vi "Terminate.vi"(8 "error in (no error)":errorcluster, 10 "Message in":refnum<class "TerminateMessage.lvclass">, 11 "ImageStack in":refnum<class "Invivo_ImageStack.lvclass">) -> (0 "error out":errorcluster, 3 "ImageStack out":refnum<class "Invivo_ImageStack.lvclass">)   [LabVIEW 2012, in "Invivo_ImageStack.lvclass"]
doc: "This member function is called when the statemachine in the run.vi receives an 'terminate' command. It closes the RabbitMQ connection. \n\nOverride this member function in your derived class to release all previously acquired resources (but don't forget to call the parent method). If your component has subcomponents, they count as resources, and you have to release them by calling their own terminate functions."
uses:
  Invivo_ImageStack.lvclass
  <vilib>/Distrio/Murmex/TerminateMessage/TerminateMessage.lvclass
  <vilib>/Distrio/Murmex/Murmex/Murmex.lvclass
panel:
  # "This method is called when the TERMINATE\ntrigger is sent. \n\nOverride this method when your component needs to\nrespond to this trigger. \n\nCall parent for proper implementation"
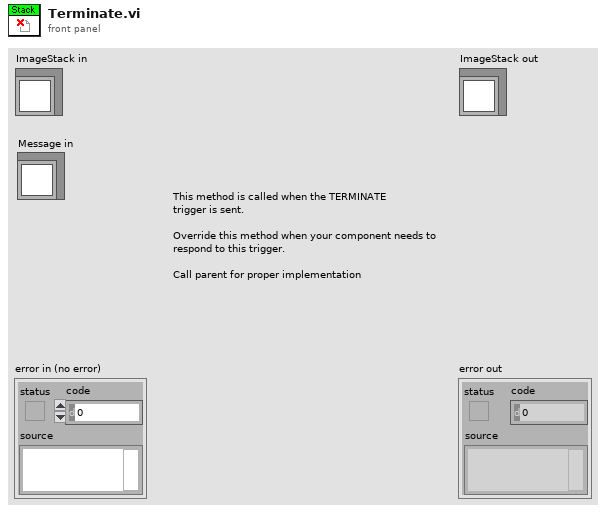
[diagram p1: front panel]
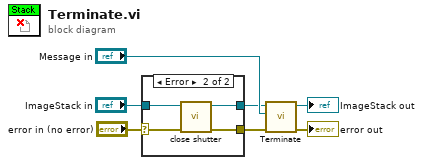
[diagram p0: block diagram]
diagram:
  n1 = case shown="Error" "error in (no error)" {
    selector: "error in (no error)" -> [w9 w13]
    tunnel: [w9 w12] -> w3
    tunnel: "ImageStack in" -> [w8 w11]
    tunnel: [w8 w10] -> w1
    frame No Error {
    }
    frame Error {
      n2 = call "close shutter.vi"("error in (no error)"=w13, "Murmex in"=w11) -> ("error out"=w12:errorcluster, "Murmex out"=w10:refnum<class "Invivo_ImageStack.lvclass">)  [unwired: 8 in]
    }
  }
  n3 = call-parent "Terminate.vi"("error in (no error)"=w3, "Message in"="Message in", "Murmex in"=w1) -> ("error out"=→"error out":errorcluster, "Murmex out"=→"ImageStack out":refnum<class "Invivo_ImageStack.lvclass">)  [unwired: 7 in]
